vi "SearchVISAResource.vi"(2 "error in":errorcluster, 3 "VISA search Expression":string="?*INSTR") -> (0 "Error list":errorcluster[](array[cluster])=[{"status"=FALSE, "code"=0, "source"=""}, {"status"=TRUE, "code"=-1073807360, "source"="VISA Open in SearchVISAResource.vi"}, {"status"=FALSE, "code"=0, "source"=""}, {"status"=TRUE, "code"=-1073807360, "source"="VISA Open in SearchVISAResource.vi"}, {"status"=TRUE, "code"=-1073807360, "source"="VISA Open in SearchVISAResource.vi"}, {"status"=TRUE, "code"=-1073807360, "source"="VISA Open in SearchVISAResource.vi"}, {"status"=TRUE, "code"=-1073807360, "source"="VISA Open in SearchVISAResource.vi"}, {"status"=TRUE, "code"=-1073807360, "source"="VISA Open in SearchVISAResource.vi"}, {"status"=TRUE, "code"=-1073807360, "source"="VISA Open in SearchVISAResource.vi"}, {"status"=TRUE, "code"=-1073807360, "source"="VISA Open in SearchVISAResource.vi"}, {"status"=TRUE, "code"=-1073807360, "source"="VISA Open in SearchVISAResource.vi"}, {"status"=TRUE, "code"=-1073807360, "source"="VISA Open in SearchVISAResource.vi"}, {"status"=TRUE, "code"=-1073807360, "source"="VISA Open in SearchVISAResource.vi"}, {"status"=TRUE, "code"=-1073807346, "source"="VISA Open in SearchVISAResource.vi"}], 1 "VISA list":refnum<visa-resource-name>[](array[refnum])=["ASRL1::INSTR", "NOEXIST", "ASRL3::INSTR", "NOEXIST", "NOEXIST", "NOEXIST", "NOEXIST", "NOEXIST", "NOEXIST", "NOEXIST", "NOEXIST", "NOEXIST", "NOEXIST", "NOEXIST"])   [LabVIEW 2012]
uses:
  <vilib>/Instr/_visa.llb/VISA Find Search Mode.ctl
panel:
  out "find list":string[](array[string])
  out "loop":i32
  out "totalSearch":i32
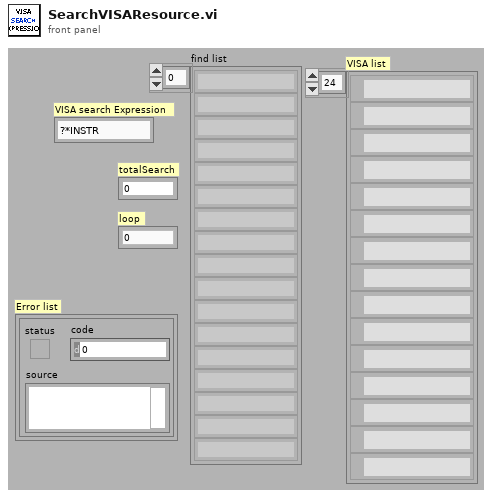
[diagram p1: front panel]
types:
  T1 = typedef "VISA Find Search Mode.ctl" = u32
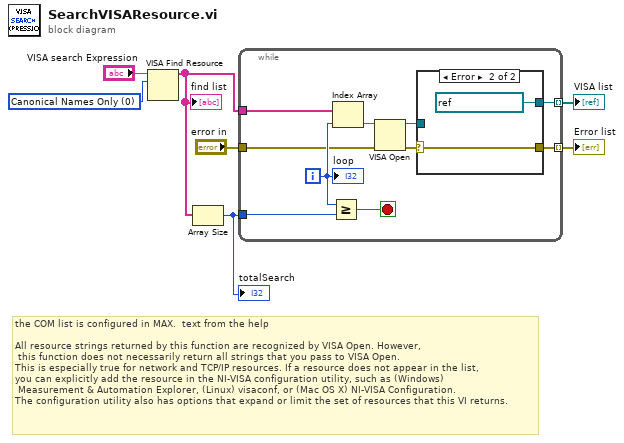
[diagram p0: block diagram]
diagram:
  w1 = T1 0 items=["Canonical Names Only"=0, "Aliases Only"=2, "Include Matching Aliases"=3, "Include All Aliases"=4] ("Search Mode")
  # "the COM list is configured in MAX.  text from the help\n\nAll resource strings returned by this function are recognized by VISA Open. However,\n this function does not necessarily return all strings that you pass to VISA Open. \nThis is especially true for network and TCP/IP resources. If a resource does not appear in the list, \nyou can explicitly add the resource in the NI-VISA configuration utility, such as (Windows)\n Measurement & Automation Explorer, (Linux) visaconf, or (Mac OS X) NI-VISA Configuration. \nThe configuration utility also has options that expand or limit the set of resources that this VI returns."
  n1 = VISA Find Resource(10:w1, 11:"VISA search Expression") -> (3:w4:string[])  [unwired: 1 in, 2 out]
  "find list" <- w4
  n2 = Array Size(array=w4) -> (size(s)=w3:i32)
  "totalSearch" <- w3
  n3 = while {
    tunnel: w4 -> [w17]
    tunnel: w3 -> [w14]
    tunnel: [w10] -> w2 mode=indexing
    tunnel: [w9] -> w6 mode=indexing
    tunnel: "error in" -> [w8]
    i -> [w15]
    stop <- w13 stop-if-true
    n4 = Greater Or Equal?(x=w15, y=w14) -> (x >= y?=w13:bool)
    n5 = Index Array(array=w17, index=w15) -> (element=w16:string)
    n6 = VISA Open(error in (no error)=w8, VISA resource name=w16) -> (VISA resource name=w11:refnum<visa-resource-name>, error out=w12:errorcluster)  [unwired: 3 in]
    n7 = case shown="Error" w12 {
      selector: w12 -> [w19 w21]
      tunnel: [w19 w21] -> w9
      tunnel: w11 -> [w18 _]
      tunnel: [w18 refnum<visa-resource-name> "NOEXIST" ("VISA resource name out")] -> w10
      frame No Error {
      }
      frame Error {
      }
    }
    "loop" <- w15
  }
  "VISA list" <- w2
  "Error list" <- w6
